vi "ReadMyConfiguration.vi"(8 "error in (no error)":errorcluster, 11 "SMO.Configurable in":refnum<class "SMO.Configurable.lvclass">) -> (0 "error out":errorcluster, 2 "Config":T1, 3 "SMO.Configurable out":refnum<class "SMO.Configurable.lvclass">)   [LabVIEW 2013, in "SMO.Configurable.lvclass"]
uses:
  SMO.Configurable.lvclass
  Config--cluster.ctl
  src/SMO/SMO.lvclass
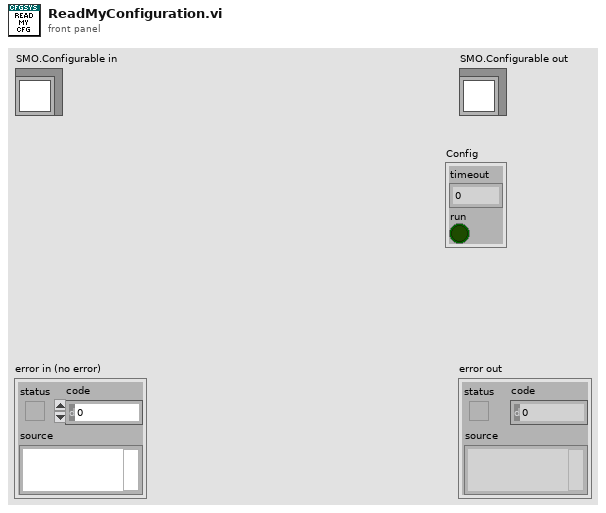
[diagram p1: front panel]
types:
  T1 = typedef "SMO.Configurable.lvclass/Config--cluster.ctl" = cluster{"timeout":i32, "run":bool}
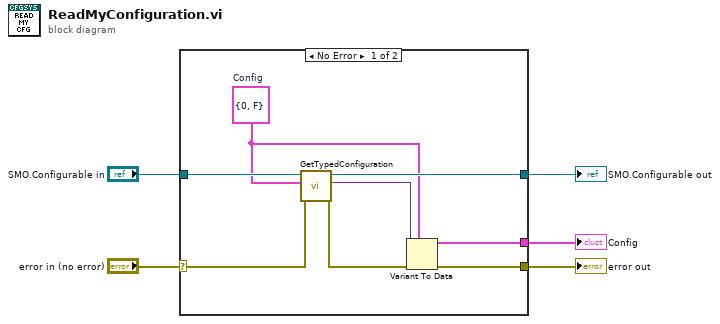
[diagram p0: block diagram]
diagram:
  n1 = case shown="No Error" "error in (no error)" {
    selector: "error in (no error)" -> [w11 w15]
    tunnel: [w6 w15] -> w4
    tunnel: [w12 w14] -> w2
    tunnel: "SMO.Configurable in" -> [w13 w14]
    tunnel: [w8 _] -> w1
    frame No Error {
      w9 = T1 {"timeout"=0, "run"=FALSE}  # Config
      n2 = call "GetTypedConfiguration.vi"("error in (no error)"=w11, "Default value"=w9, "SMO"=w13) -> ("error out"=w7:errorcluster, "Variant"=w10:variant, "SMO out"=w12:refnum<class "SMO.Configurable.lvclass">)  [unwired: 4 in, 2 out]
      n3 = Variant To Data(error in=w7, type=w9, Variant=w10) -> (data=w8:T1, error out=w6:errorcluster)
    }
    frame Error {
    }
  }
  "error out" <- w4
  "SMO.Configurable out" <- w2
  "Config" <- w1
